vi "svfa_Average Spectrum (complex) No State.vi"(0 "spectrum":cluster{"f0":dbl, "df":dbl, "spectrum":cdb[]} {"spectrum" format="%.2p"; "df" format="%.2p"; "f0" format="%.2p"}, 1 "processing control":T1(ring), 7 "averaging parameters":T3={"averaging mode"=enum."No averaging", "weighting mode"=enum."Linear", "number of averages"=10, "linear mode"=enum."Auto restart"}, 11 "error in (no error)":errorcluster, 12 "averaging state info in":T2={"complex FFT"=[], "real FFT"=[], "f0"=0.0, "df"=0.0, "averages completed"=0.0, "averaging parameters"={"averaging mode"=enum."No averaging", "weighting mode"=enum."Linear", "number of averages"=10, "linear mode"=enum."Auto restart"}} {"averages completed" format="%.2f"; "df" format="%.2f"; "f0" format="%.2f"; "real FFT" format="%.2f"; "complex FFT" format="%.2f"}) -> (4 "average spectrum":cluster{"f0":dbl, "df":dbl, "spectrum":cdb[]} {"spectrum" format="%.2p"; "df" format="%.2p"; "f0" format="%.2p"}, 6 "new spectrum ready":bool, 8 "averaging done":bool, 10 "averages completed":dbl, 14 "averaging state info out":T2={"complex FFT"=[], "real FFT"=[], "f0"=0.0, "df"=0.0, "averages completed"=0.0, "averaging parameters"={"averaging mode"=enum."No averaging", "weighting mode"=enum."Linear", "number of averages"=10, "linear mode"=enum."Auto restart"}} {"averages completed" format="%.2f"; "df" format="%.2f"; "f0" format="%.2f"; "real FFT" format="%.2f"; "complex FFT" format="%.2f"}, 15 "error out":errorcluster)   [LabVIEW 2017]
uses:
  <vilib>/addons/_NISVFA/_Shared subVIs/Spectrum Averaging/svfa_Average Array (complex) No State.vi
  <vilib>/addons/_NISVFA/_Shared subVIs/Spectrum Averaging/svfa_No Average Array (complex).vi
  <vilib>/addons/_NISVFA/_Shared subVIs/Spectrum Averaging/svfa_Average Array (complex).vi
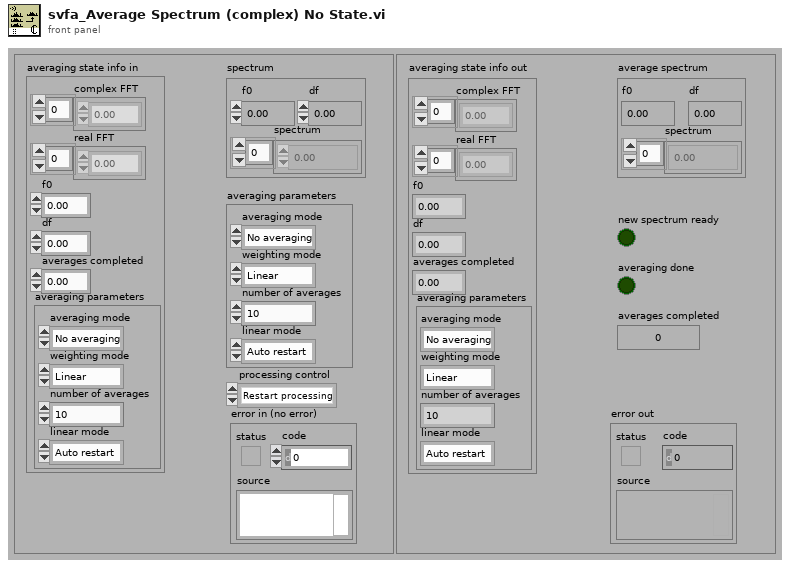
[diagram p1: front panel]
types:
  T1 = enum16{"Restart processing", "Continue processing", "Skip processing"}
  T2 = cluster{"complex FFT":cdb[], "real FFT":dbl[], "f0":dbl, "df":dbl, "averages completed":dbl, "averaging parameters":cluster{"averaging mode":enum16{"No averaging", "Vector averaging", "RMS averaging", "Peak hold"}, "weighting mode":enum16{"Linear", "Exponential"}, "number of averages":u32, "linear mode":enum16{"One shot", "Auto restart"}}}
  T3 = cluster{"averaging mode":enum16{"No averaging", "Vector averaging", "RMS averaging", "Peak hold"}, "weighting mode":enum16{"Linear", "Exponential"}, "number of averages":u32, "linear mode":enum16{"One shot", "Auto restart"}}
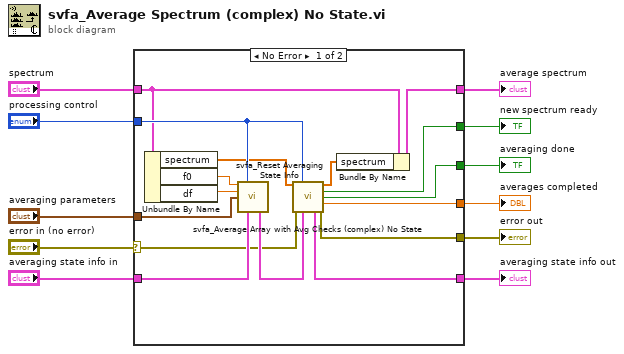
[diagram p0: block diagram]
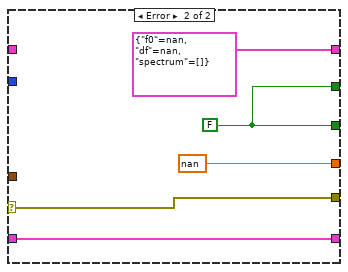
[diagram p2: hidden frame]
diagram:
  n1 = case shown="No Error" "error in (no error)" {
    selector: "error in (no error)" -> [w18 w32]
    tunnel: "averaging parameters" -> [w14 _]
    tunnel: [w26 w29] -> w5
    tunnel: [w27 w29] -> w3
    tunnel: [w25 nan ("f0")] -> w11
    tunnel: "spectrum" -> [w13 _]
    tunnel: "averaging state info in" -> [w21 w31]
    tunnel: [w24 w31] -> w2
    tunnel: [w23 cluster{"f0":dbl, "df":dbl, "spectrum":cdb[]} {"f0"=nan, "df"=nan, "spectrum"=[]} ("dup spectrum")] -> w10
    tunnel: "processing control" -> [w22 _]
    tunnel: [w19 w32] -> w4
    frame No Error {
      n2 = Unbundle By Name(w13) -> ("spectrum"=w17:cdb[], "f0"=w15:dbl, "df"=w16:dbl)
      n3 = call <vilib>:"svfa_Reset Averaging State Info.vi"("f0"=w15, "processing control"=w22, "df"=w16, "averaging parameters"=w14, "averaging state info in"=w21) -> ("averaging state info out"=w20:T2)  [unwired: 9 in, 1 out]
      n4 = call <vilib>:"svfa_Average Array with Avg Checks (complex) No State.vi"("spectrum"=w17, "processing control"=w22, "error in (no error)"=w18, "averaging state info in"=w20) -> ("average spectrum"=w12:cdb[], "new spectrum ready"=w27:bool, "averaging done"=w26:bool, "averages completed"=w25:dbl, "averaging state info out"=w24:T2, "error out"=w19:errorcluster)  [unwired: 6 in]
      n5 = Bundle By Name(cluster=w13, "spectrum"=w12) -> (w23:cluster{"f0":dbl, "df":dbl, "spectrum":cdb[]})
    }
    frame Error {
      w29 = FALSE
    }
  }
  "averages completed" <- w11
  "average spectrum" <- w10
  "averaging done" <- w5
  "error out" <- w4
  "new spectrum ready" <- w3
  "averaging state info out" <- w2
